vi "TagBrowse.vi"(7 "LabVIEW Web Service Request":refnum<class "Web Request.lvclass">) -> ()   [LabVIEW 2013]
doc: "TagBrowse returns a list of the name, type, and permissions of every tag in the CVT."
uses:
  <vilib>/wsapi/Web Request.lvclass
  <vilib>/NI/Tag Bus Module Framework/channel/TBM channel.lvclass
  <vilib>/NI/TagWebClient/API/JSON Formats/TagBrowse Results.ctl
  <vilib>/NI/TagWebClient/API/Logical Groups/Tags in Group.ctl
  <vilib>/NI/TagWebClient/API/Logical Groups/tags.ctl
  <vilib>/NI/Tag Bus/tag/tag descriptor.lvclass/tag descriptor.ctl
  <vilib>/NI/Tag Bus Module Framework/channel/TBM channel.lvclass/TBM channel.ctl
  <vilib>/NI/Tag Bus/tag/read tag name.vi
  <vilib>/NI/Tag Bus Module Framework/channel/Read channel classification.vi
  <vilib>/NI/Tag Bus/tag/count types.vi
  <vilib>/NI/Tag Bus/tag/index to type.vi
  <vilib>/NI/TagWebClient/API/tagweb client API.lvlib
  <vilib>/NI/Tag Bus/tag/tag descriptor.lvclass
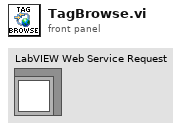
[diagram p1: front panel]
types:
  T1 = typedef "tagweb client API.lvlib/TagBrowse Results.ctl" = cluster{"groupName":string, "Tags":T2[]}
  T2 = typedef "tagweb client API.lvlib/Tags in Group.ctl" = cluster{"type":string, "tags":T3[]}
  T3 = typedef "tagweb client API.lvlib/tags.ctl" = cluster{"tagName":string, "permissions":string}
  T4 = typedef "tag bus.lvlib/tag descriptor.lvclass/Data Type.ctl" = enum16{"Double", "Single", "I64", "I32", "I16", "I8", "U64", "U32", "U16", "U8", "Boolean", "String", "Array of Double", "Array of Single", "Array of I64", "Array of I32", "Array of I16", "Array of I8", "Array of U64", "Array of U32", "Array of U16", "Array of U8", "Array of Boolean", "Array of String"}
  T5 = typedef "TBM channel.lvclass/channel classification.ctl" = enum16{"input data", "output data", "processing parameter", "processing result"}
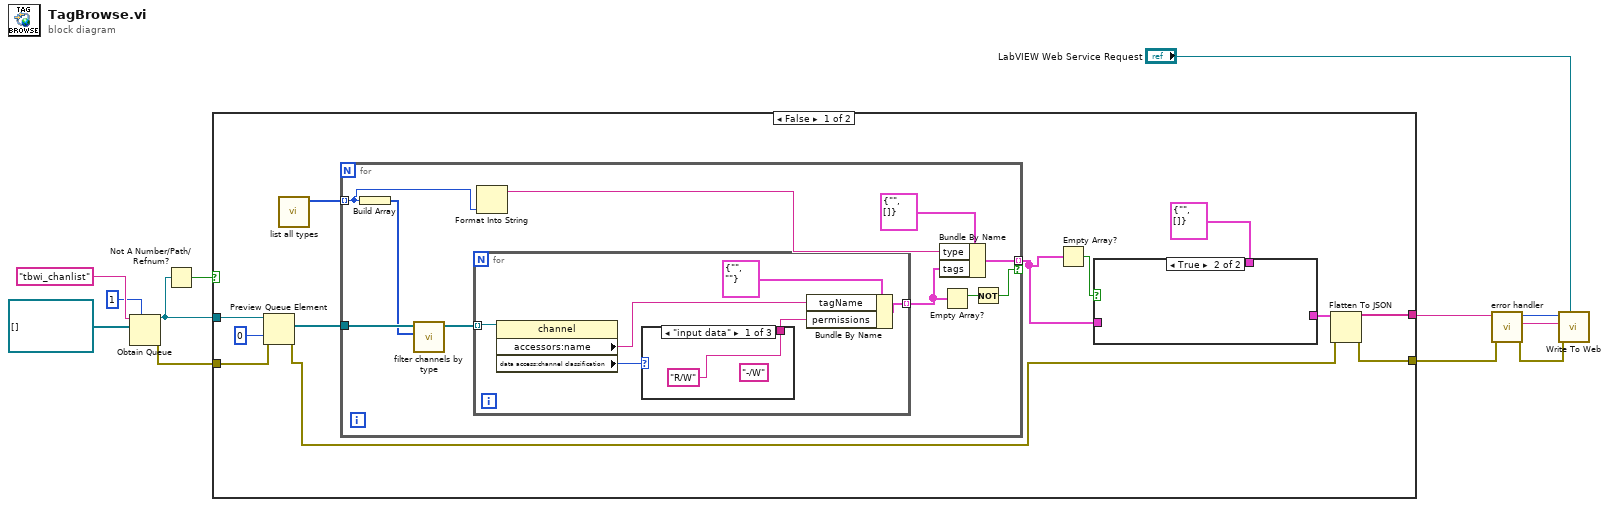
[diagram p0: block diagram]
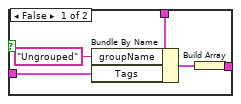
[diagram p2: hidden frame]
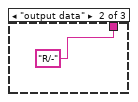
[diagram p3: hidden frame]
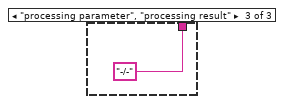
[diagram p4: hidden frame]
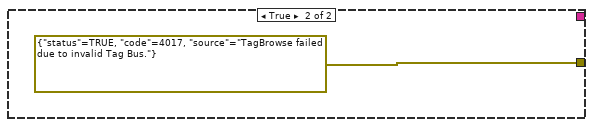
[diagram p5: hidden frame]
diagram:
  n1 = Obtain Queue(max queue size (-1, unlimited)=1, name (unnamed)="tbwi_chanlist", element data type=refnum<class "TBM channel.lvclass">[] [] ("channels in")) -> (queue out=w3:refnum<queue>, error out=w4:errorcluster)  [unwired: 2 in, 1 out]
  n2 = Not A Number/Path/Refnum?(number/path/refnum=w3) -> (NaN/Path/Refnum?=w2:bool)
  n3 = case shown="False" w2 {
    tunnel: w4 -> [w24 _]
    tunnel: w3 -> [w23 _]
    tunnel: [w19 errorcluster {"status"=TRUE, "code"=4017, "source"="TagBrowse failed due to invalid Tag Bus."} ("error out")] -> w12
    tunnel: [w20 _] -> w11
    frame False {
      n4 = Preview Queue Element(queue=w23, timeout in ms (-1)=0, error in (no error)=w24) -> (element=w16:refnum<class "TBM channel.lvclass">[], error out=w18:errorcluster)  [unwired: 2 out]
      n5 = call <vilib>:"list all types.vi"() -> ("all types"=w17:T4[])  [unwired: 11 in]
      n6 = for {
        tunnel: w17 -> [w39] mode=indexing
        tunnel: w16 -> [w36]
        tunnel: [w37] -> w14 mode=indexing if=w31
        n7 = Build Array(w39) -> (w34:T4[])
        n8 = call <vilib>:"filter channels by type.vi"("allowed types"=w34, "channels in"=w36) -> ("channels out"=w35:refnum<class "TBM channel.lvclass">[])  [unwired: 9 in]
        n9 = for {
          tunnel: [w45] -> w33 mode=indexing
          tunnel: w35 -> [w44] mode=indexing
          n10 = property class="channel"(reference=w44) -> ("accessors:name"=w43:string, "data access:channel classification"=w42:T5)  [unwired: 1 in, 2 out]
          n11 = case shown="\"input data\"" w42 {
            tunnel: ["R/W" "R/-" "-/-"] -> w41
            frame "input data" {
              (unwired) "-/W"
            }
            frame "output data" {
            }
            frame "processing parameter", "processing result" {
            }
          }
          n12 = Bundle By Name(cluster=T3 {"tagName"="", "permissions"=""} ("tags"), "tagName"=w43, "permissions"=w41) -> (w45:T3)
        }
        n13 = Format Into String(w39) -> (resulting string=w38:string)  [unwired: 3 in, 1 out]
        n14 = Bundle By Name(cluster=T2 {"type"="", "tags"=[]} ("Cluster"), "type"=w38, "tags"=w33) -> (w37:T2)
        n15 = Empty Array?(array=w33) -> (empty?=w32:bool)
        n16 = Not(x=w32) -> (.not. x?=w31:bool)
      }
      n17 = Empty Array?(array=w14) -> (empty?=w13:bool)
      n18 = case shown="True" w13 {
        tunnel: [w27 _] -> w21
        tunnel: T1 {"groupName"="", "Tags"=[]} ("TagBrowse Results") -> [w26 _]
        tunnel: w14 -> [w25 _]
        frame False {
          n19 = Bundle By Name(cluster=w26, "groupName"="Ungrouped", "Tags"=w25) -> (w28:T1)
          n20 = Build Array(w28) -> (w27:T1[])
        }
        frame True {
        }
      }
      n21 = Flatten To JSON(anything=w21, error in (no error)=w18) -> (JSON string=w20:string, 11:w19:errorcluster)  [unwired: 1 in]
    }
    frame True {
    }
  }
  n22 = call "error handler.vi"("error in (no error)"=w12, "Success Message"=w11) -> ("error out"=w10:errorcluster, "Response String"=w8:string, "Response Code"=w9:i32)  [unwired: 7 in]
  n23 = call <vilib>:"Write To Web.vi"("Web Request in"="LabVIEW Web Service Request", "error in"=w10, "Response String"=w8, "Response Code"=w9) -> ()  [unwired: 8 in]
